vi "combine_time_and_counts.vi"(10 "Voltage In":dbl[][](array[numeric]), 11 "Time":dbl[](array[numeric])) -> (3 "Traces Out":dbl[][][](array[numeric]))   [LabVIEW 2016]
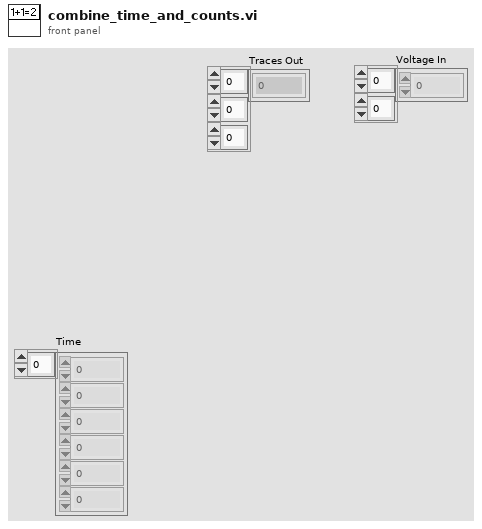
[diagram p1: front panel]
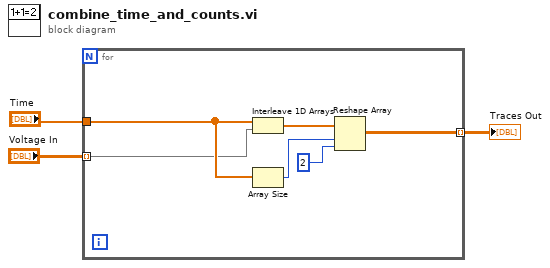
[diagram p0: block diagram]
diagram:
  n1 = for {
    tunnel: "Time" -> [w8]
    tunnel: [w5] -> w1 mode=indexing
    tunnel: "Voltage In" -> [w4] mode=indexing
    n2 = Interleave 1D Arrays(w8, w4) -> (w9:dbl[])
    n3 = Array Size(array=w8) -> (size(s)=w7:i32)
    n4 = Reshape Array(w9, w7, 2 ("dimension size")) -> (w5:dbl[][])
  }
  "Traces Out" <- w1
